vi "RichToFlatcif_manager_LoaderDestroy.vi"(5 "OutputClusterType":T1, 11 "InputCluster":T2) -> (3 "OutputCluster":T1)   [LabVIEW 2021, in "CIF_PluginLoader_client.lvlib"]
uses:
  CIF_PluginLoader_client.lvlib
  cif_manager_LoaderDestroy.ctl
  cif_manager_LoaderDestroy_Flat.ctl
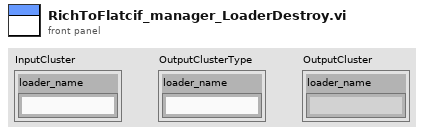
[diagram p1: front panel]
types:
  T1 = typedef "CIF_PluginLoader_client.lvlib/cif_manager_LoaderDestroy_Flat.ctl" = cluster{"loader_name":string}
  T2 = typedef "CIF_PluginLoader_client.lvlib/cif_manager_LoaderDestroy.ctl" = cluster{"loader_name":string}
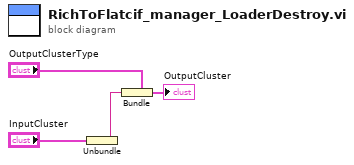
[diagram p0: block diagram]
diagram:
  n1 = Unbundle "Unbundle"("InputCluster") -> ("loader_name"=w1:string)
  n2 = Bundle "Bundle"(cluster="OutputClusterType", "loader_name"=w1) -> (→"OutputCluster":T1)
